vi "PopAll.vi"(11 "POTTypedCircularBuffer in":refnum<class "ErrorLogBuffer.lvclass">) -> (2 "Flushed Buffer":T1[](array[typedef]), 3 "POTTypedCircularBuffer out":refnum<class "ErrorLogBuffer.lvclass">)   [LabVIEW 2024, in "ErrorLogBuffer.lvclass"]
uses:
  ErrorLogBuffer.lvclass
  Type.ctl
  RQMHCore/ErrorReporting/Record/LogRecord.lvclass
  ErrorLogBuffer.lvclass/ErrorLogBuffer.ctl
  ReadCount.vi
  Reorder.vi
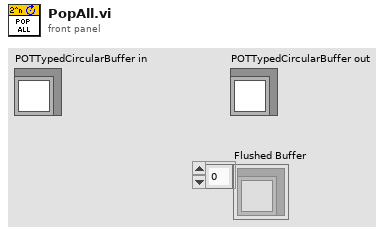
[diagram p1: front panel]
types:
  T1 = typedef "ErrorLogBuffer.lvclass/Type.ctl" = refnum<class "LogRecord.lvclass">
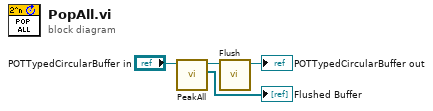
[diagram p0: block diagram]
diagram:
  n1 = call "PeakAll.vi"("POTTypedCircularBuffer in"="POTTypedCircularBuffer in") -> ("Copied Buffer"=→"Flushed Buffer":T1[], "POTTypedCircularBuffer out"=w4:refnum<class "ErrorLogBuffer.lvclass">)  [unwired: 9 in]
  n2 = call "Flush.vi"("POTTypedCircularBuffer in"=w4) -> ("POTTypedCircularBuffer out"=→"POTTypedCircularBuffer out":refnum<class "ErrorLogBuffer.lvclass">)  [unwired: 10 in]
